vi "ConfigUtilities - Set Rx Channels.vi"(8 "error in (no error)":errorcluster, 9 "Rx Channel Paths":string[](array[string]), 10 "Rx Channel Names":string[](array[string]), 11 "Item Ref in":T1 format="%.0x") -> (0 "error out":errorcluster, 3 "Item Ref out":T1=18446744073709551615 format="%.0x")   [LabVIEW 2016, in "UDP-Custom-Device System Explorer.lvlib"]
uses:
  UDP-Custom-Device System Explorer.lvlib
  <vilib>/NI Veristand/Custom Device API/Custom Device Item Ref.ctl
  Shared/Constants.vi
  <vilib>/NI Veristand/Custom Device API/Get Item Property (Dependent Node Pointer).vi
  <vilib>/NI VeriStand/Custom Device Tools/Custom Device Utility Library/Custom Device Utility Library.lvlib
  <vilib>/NI VeriStand/Custom Device API/Custom Device API.lvlib
  Shared/UDP-Custom-Device Shared.lvlib
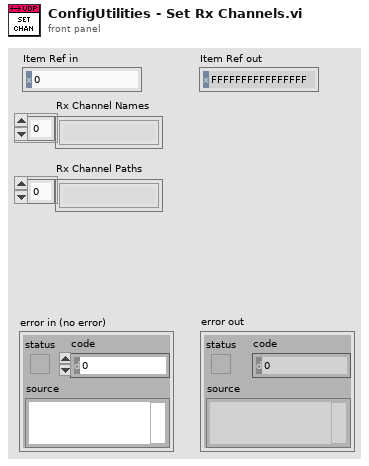
[diagram p1: front panel]
types:
  T1 = typedef "Custom Device API.lvlib/Custom Device Item Ref.ctl" = u64
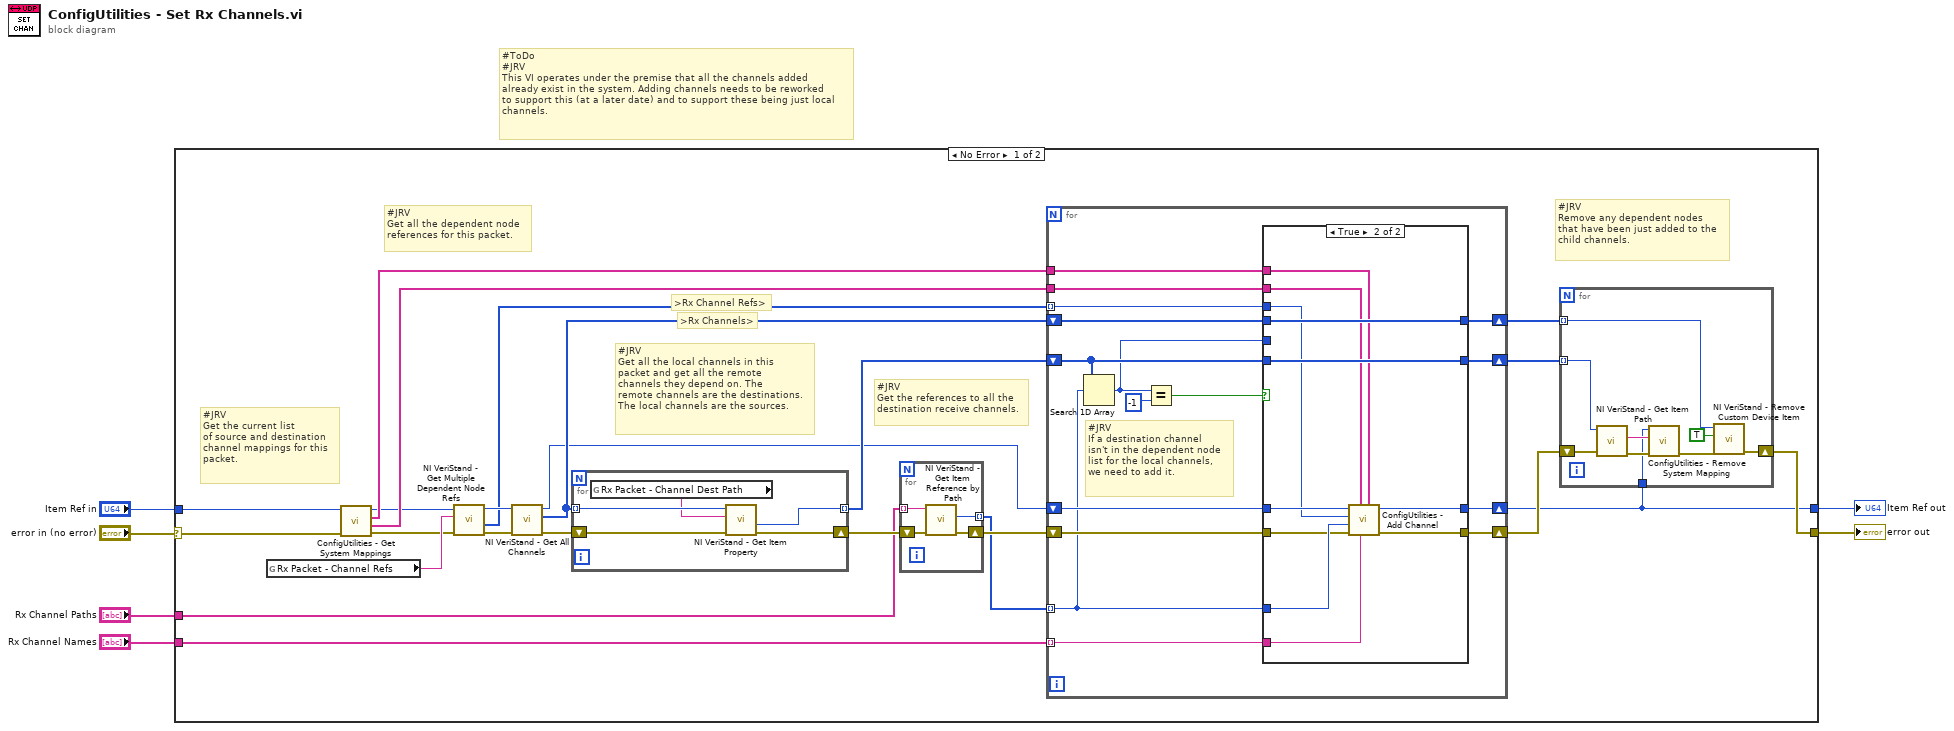
[diagram p0: block diagram]
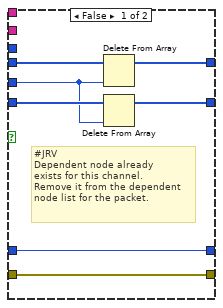
[diagram p2: hidden frame]
diagram:
  # "#ToDo\n#JRV\nThis VI operates under the premise that all the channels added\nalready exist in the system. Adding channels needs to be reworked\nto support this (at a later date) and to support these being just local\nchannels."
  n1 = case shown="No Error" "error in (no error)" {
    selector: "error in (no error)" -> [w16 w83]
    tunnel: "Item Ref in" -> [w13 w84]
    tunnel: [w12 w84] -> w4
    tunnel: [w25 w83] -> w3
    tunnel: "Rx Channel Paths" -> [w8 _]
    tunnel: "Rx Channel Names" -> [w7 _]
    frame No Error {
      # "#JRV\nRemove any dependent nodes\nthat have been just added to the\nchild channels."
      # "#JRV\nGet the references to all the\ndestination receive channels."
      # "#JRV\nGet all the local channels in this\npacket and get all the remote \nchannels they depend on. The\nremote channels are the destinations.\nThe local channels are the sources."
      # "#JRV\nGet all the dependent node\nreferences for this packet."
      # "#JRV\nGet the current list\nof source and destination\nchannel mappings for this\npacket."
      # ">Rx Channels>"
      # ">Rx Channel Refs>"
      n2 = global read "Constants.vi" "Rx Packet - Channel Refs"() -> (w19:string)
      n3 = call "ConfigUtilities - Get System Mappings.vi"("error in (no error)"=w16, "Item Ref in"=w13) -> ("error out"=w14:errorcluster, "Channel Path Destinations"=w17:string[], "Channel Path Sources"=w18:string[], "Item Ref out"=w15:T1)  [unwired: 6 in]
      n4 = call <vilib>:"NI VeriStand - Get Multiple Dependent Node Refs.vi"("error in (no error)"=w14, "Base Property Name"=w19, "Item Ref in"=w15) -> ("error out"=w29:errorcluster, "Dependent Node Refs"=w10:T1[], "Item Ref out"=w28:T1)  [unwired: 6 in]
      n5 = call <vilib>:"NI VeriStand - Get All Channels.vi"("error in"=w29, "Section Ref in"=w28) -> ("error out"=w30:errorcluster, "Channel Refs"=w27:T1[], "Section Ref out"=w11:T1)  [unwired: 6 in, 1 out]
      n6 = for {
        tunnel: w27 -> [w82] mode=indexing
        tunnel: [w80] -> w23 mode=indexing
        shift-right: [w79] -> w22
        shift-left: w30 -> [w81]
        n7 = global read "Constants.vi" "Rx Packet - Channel Dest Path"() -> (w78:string)
        n8 = call-poly <vilib>:"NI VeriStand - Get Item Property.vi"("error in (no error)"=w81, "Property Name"=w78, "Item Ref in"=w82) -> ("error out"=w79:errorcluster, "Dependent Node Ref"=w80:T1)  [unwired: 5 in, 2 out]
      }
      n9 = for {
        tunnel: w8 -> [w77] mode=indexing
        tunnel: [w76] -> w9 mode=indexing
        shift-right: [w74] -> w21
        shift-left: w22 -> [w75]
        n10 = call <vilib>:"NI VeriStand - Get Item Reference by Path.vi"("error in (no error)"=w75, "Item Path in"=w77) -> ("error out"=w74:errorcluster, "Item Ref"=w76:T1)  [unwired: 6 in, 2 out]
      }
      n11 = for {
        tunnel: w9 -> [w41] mode=indexing
        shift-right: [w40] -> w26
        shift-left: w21 -> [w44]
        tunnel: w7 -> [w42] mode=indexing
        tunnel: w10 -> [w39] mode=indexing
        shift-right: [w36] -> w24
        shift-left: w27 -> [w37]
        shift-right: [w34] -> w20
        shift-left: w23 -> [w35]
        tunnel: w18 -> [w31]
        tunnel: w17 -> [w32]
        shift-right: [w38] -> w12
        shift-left: w11 -> [w43]
        # "#JRV\nIf a destination channel\nisn't in the dependent node\nlist for the local channels,\nwe need to add it."
        n12 = Search 1D Array(1D array=w35, element=w41) -> (index of element=w33:i32)  [unwired: 1 in]
        n13 = Equal?(x=w33, y=-1) -> (x = y?=w45:bool)
        n14 = case shown="True" w45 {
          tunnel: w44 -> [w48 w59]
          tunnel: w43 -> [w47 w56]
          tunnel: w42 -> [_ w57]
          tunnel: w41 -> [_ w60]
          tunnel: [w48 w58] -> w40
          tunnel: w39 -> [_ w54]
          tunnel: [w47 w55] -> w38
          tunnel: w37 -> [w53 w64]
          tunnel: [w52 w64] -> w36
          tunnel: w33 -> [w49 _]
          tunnel: w35 -> [w51 w63]
          tunnel: [w50 w63] -> w34
          tunnel: w32 -> [_ w62]
          tunnel: w31 -> [_ w61]
          frame False {
            # "#JRV\nDependent node already\nexists for this channel.\nRemove it from the dependent\nnode list for the packet."
            n15 = Delete From Array(array=w53, index=w49) -> (array with subset deleted=w52:T1[])  [unwired: 1 in, 1 out]
            n16 = Delete From Array(array=w51, index=w49) -> (array with subset deleted=w50:T1[])  [unwired: 1 in, 1 out]
          }
          frame True {
            n17 = call "ConfigUtilities - Add Channel.vi"("Channel Path Sources"=w61, "Rx Channel Name"=w57, "Channel Path Destinations"=w62, "error in (no error)"=w59, "Rx Channel Ref"=w60, "Dependent Node Ref"=w54, "Rx Section Ref in"=w56) -> ("error out"=w58:errorcluster, "Rx Section Ref in"=w55:T1)  [unwired: 3 in]
          }
        }
      }
      n18 = for {
        shift-right: [w73] -> w25
        shift-left: w26 -> [w71]
        tunnel: w24 -> [w66] mode=indexing
        tunnel: w20 -> [w67] mode=indexing
        tunnel: w12 -> [w65]
        n19 = call <vilib>:"NI VeriStand - Get Item Path.vi"("error in (no error)"=w71, "Item Ref in"=w67) -> ("error out"=w70:errorcluster, "Path"=w68:string)  [unwired: 6 in, 2 out]
        n20 = call "ConfigUtilities - Remove System Mapping.vi"("error in (no error)"=w70, "Channel Path Destination"=w68, "Item Ref in"=w65) -> ("error out"=w69:errorcluster)  [unwired: 7 in, 1 out]
        n21 = call <vilib>:"NI VeriStand - Remove Custom Device Item.vi"("error in (no error)"=w69, "Force Delete (F)"=TRUE, "Item Ref in"=w66) -> ("error out"=w73:errorcluster)  [unwired: 7 in, 1 out]
      }
    }
    frame Error {
    }
  }
  "Item Ref out" <- w4
  "error out" <- w3
